vi "System Options.vi"(8 "error in":errorcluster, 9 "Beeper Mode (1:Beep on Pass)":i32(ring)=1 items=["No Beep", "Beep on Pass", "Beep on Fail"], 10 "Display Mode (1:On)":i32(ring)=1 items=["Off", "On"], 11 "VISA resource name":refnum<visa-resource-name>) -> (0 "error out":errorcluster, 3 "VISA resource name out":refnum<visa-resource-name>)   [LabVIEW 2021, in "GWInstek  GDM8351.lvlib"]
doc: "Sets the display status and beeper mode."
uses:
  <instrlib>/GWInstek  GDM8351/GWInstek  GDM8351.lvlib
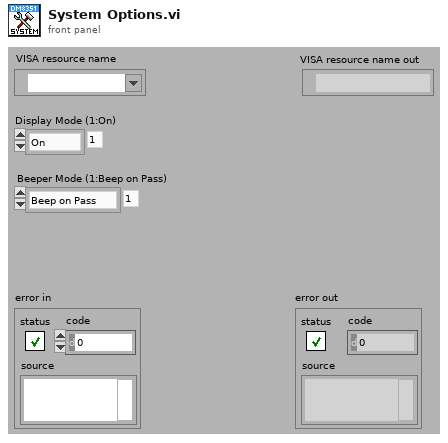
[diagram p1: front panel]
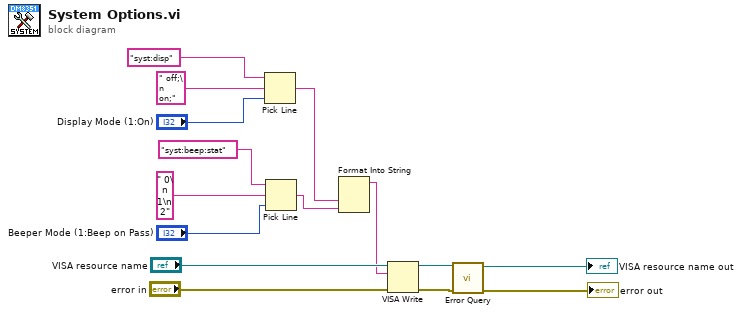
[diagram p0: block diagram]
diagram:
  n1 = Pick Line(string ("")="syst:disp", multi-line string=" off;\n on;", line index="Display Mode (1:On)") -> (output string=w2:string)
  n2 = Pick Line(string ("")="syst:beep:stat", multi-line string=" 0\n 1\n 2", line index="Beeper Mode (1:Beep on Pass)") -> (output string=w3:string)
  n3 = Format Into String(w2, w3) -> (resulting string=w1:string)  [unwired: 3 in, 1 out]
  n4 = VISA Write(VISA resource name="VISA resource name", write buffer=w1, error in (no error)="error in") -> (VISA resource name out=w7:refnum<visa-resource-name>, error out=w6:errorcluster)  [unwired: 1 out]
  n5 = call <instrlib>:"Error Query.vi"("error in (no error)"=w6, "VISA resource name"=w7) -> ("error out"=→"error out":errorcluster, "VISA resource name out"=→"VISA resource name out":refnum<visa-resource-name>)  [unwired: 6 in, 2 out]
